vi "ProfilerTest.vi"() -> ()   [LabVIEW 2014] (continued)
"delVelocity"=0.0}, {"Time"=19.800000000000296, "delVelocity"=0.0}, {"Time"=19.810000000000297, "delVelocity"=0.0}, {"Time"=19.8200000000003, "delVelocity"=0.0}, {"Time"=19.8300000000003, "delVelocity"=0.0}, {"Time"=19.840000000000302, "delVelocity"=0.0}, {"Time"=19.850000000000303, "delVelocity"=0.0}, {"Time"=19.860000000000305, "delVelocity"=0.0}, {"Time"=19.870000000000307, "delVelocity"=0.0}, {"Time"=19.880000000000308, "delVelocity"=0.0}, {"Time"=19.89000000000031, "delVelocity"=0.0}, {"Time"=19.90000000000031, "delVelocity"=0.0}, {"Time"=19.910000000000313, "delVelocity"=0.0}, {"Time"=19.920000000000314, "delVelocity"=0.0}, {"Time"=19.930000000000316, "delVelocity"=0.0}, {"Time"=19.940000000000317, "delVelocity"=0.0}, {"Time"=19.95000000000032, "delVelocity"=0.0}, {"Time"=19.96000000000032, "delVelocity"=0.0}, {"Time"=19.970000000000322, "delVelocity"=0.0}, {"Time"=19.980000000000324, "delVelocity"=0.0}, {"Time"=19.990000000000325, "delVelocity"=0.0}, {"Time"=20.000000000000327, "delVelocity"=0.0}, {"Time"=20.01000000000033, "delVelocity"=0.0}, {"Time"=20.02000000000033, "delVelocity"=0.0}, {"Time"=20.03000000000033, "delVelocity"=0.0}, {"Time"=20.040000000000333, "delVelocity"=0.0}, {"Time"=20.050000000000335, "delVelocity"=0.0}, {"Time"=20.060000000000336, "delVelocity"=0.0}, {"Time"=20.070000000000338, "delVelocity"=0.0}, {"Time"=20.08000000000034, "delVelocity"=0.0}, {"Time"=20.09000000000034, "delVelocity"=0.0}, {"Time"=20.100000000000342, "delVelocity"=0.0}, {"Time"=20.110000000000344, "delVelocity"=0.0}, {"Time"=20.120000000000346, "delVelocity"=0.0}, {"Time"=20.130000000000347, "delVelocity"=0.0}, {"Time"=20.14000000000035, "delVelocity"=0.0}, {"Time"=20.15000000000035, "delVelocity"=0.0}, {"Time"=20.160000000000352, "delVelocity"=0.0}, {"Time"=20.170000000000353, "delVelocity"=0.0}, {"Time"=20.180000000000355, "delVelocity"=0.0}, {"Time"=20.190000000000357, "delVelocity"=0.0}, {"Time"=20.200000000000358, "delVelocity"=0.0}, {"Time"=20.21000000000036, "delVelocity"=0.0}, {"Time"=20.22000000000036, "delVelocity"=0.0}, {"Time"=20.230000000000363, "delVelocity"=0.0}, {"Time"=20.240000000000364, "delVelocity"=0.0}, {"Time"=20.250000000000366, "delVelocity"=0.0}, {"Time"=20.260000000000367, "delVelocity"=0.0}, {"Time"=20.27000000000037, "delVelocity"=0.0}, {"Time"=20.28000000000037, "delVelocity"=0.0}, {"Time"=20.290000000000372, "delVelocity"=0.0}, {"Time"=20.300000000000374, "delVelocity"=0.0}, {"Time"=20.310000000000375, "delVelocity"=0.0}, {"Time"=20.320000000000377, "delVelocity"=0.0}, {"Time"=20.33000000000038, "delVelocity"=0.0}, {"Time"=20.34000000000038, "delVelocity"=0.0}, {"Time"=20.35000000000038, "delVelocity"=0.0}, {"Time"=20.360000000000383, "delVelocity"=0.0}, {"Time"=20.370000000000385, "delVelocity"=0.0}, {"Time"=20.380000000000386, "delVelocity"=0.0}, {"Time"=20.390000000000388, "delVelocity"=0.0}, {"Time"=20.40000000000039, "delVelocity"=0.0}, {"Time"=20.41000000000039, "delVelocity"=0.0}, {"Time"=20.420000000000393, "delVelocity"=0.0}, {"Time"=20.430000000000394, "delVelocity"=0.0}, {"Time"=20.440000000000396, "delVelocity"=0.0}, {"Time"=20.450000000000397, "delVelocity"=0.0}, {"Time"=20.4600000000004, "delVelocity"=0.0}, {"Time"=20.4700000000004, "delVelocity"=0.0}, {"Time"=20.480000000000402, "delVelocity"=0.0}, {"Time"=20.490000000000403, "delVelocity"=0.0}, {"Time"=20.500000000000405, "delVelocity"=0.0}, {"Time"=20.510000000000407, "delVelocity"=0.0}, {"Time"=20.520000000000408, "delVelocity"=0.0}, {"Time"=20.53000000000041, "delVelocity"=0.0}, {"Time"=20.54000000000041, "delVelocity"=0.0}, {"Time"=20.550000000000413, "delVelocity"=0.0}, {"Time"=20.560000000000414, "delVelocity"=0.0}, {"Time"=20.570000000000416, "delVelocity"=0.0}, {"Time"=20.580000000000418, "delVelocity"=0.0}, {"Time"=20.59000000000042, "delVelocity"=0.0}, {"Time"=20.60000000000042, "delVelocity"=0.0}, {"Time"=20.610000000000422, "delVelocity"=0.0}, {"Time"=20.620000000000424, "delVelocity"=0.0}, {"Time"=20.630000000000425, "delVelocity"=0.0}, {"Time"=20.640000000000427, "delVelocity"=0.0}, {"Time"=20.65000000000043, "delVelocity"=0.0}, {"Time"=20.66000000000043, "delVelocity"=0.0}, {"Time"=20.67000000000043, "delVelocity"=0.0}, {"Time"=20.680000000000433, "delVelocity"=0.0}, {"Time"=20.690000000000435, "delVelocity"=0.0}, {"Time"=20.700000000000436, "delVelocity"=0.0}, {"Time"=20.710000000000438, "delVelocity"=0.0}, {"Time"=20.72000000000044, "delVelocity"=0.0}, {"Time"=20.73000000000044, "delVelocity"=0.0}, {"Time"=20.740000000000443, "delVelocity"=0.0}, {"Time"=20.750000000000444, "delVelocity"=0.0}, {"Time"=20.760000000000446, "delVelocity"=0.0}, {"Time"=20.770000000000447, "delVelocity"=0.0}, {"Time"=20.78000000000045, "delVelocity"=0.0}, {"Time"=20.79000000000045, "delVelocity"=0.0}, {"Time"=20.800000000000452, "delVelocity"=0.0}, {"Time"=20.810000000000453, "delVelocity"=0.0}, {"Time"=20.820000000000455, "delVelocity"=0.0}, {"Time"=20.830000000000457, "delVelocity"=0.0}, {"Time"=20.840000000000458, "delVelocity"=0.0}, {"Time"=20.85000000000046, "delVelocity"=0.0}, {"Time"=20.86000000000046, "delVelocity"=0.0}, {"Time"=20.870000000000463, "delVelocity"=0.0}, {"Time"=20.880000000000464, "delVelocity"=0.0}, {"Time"=20.890000000000466, "delVelocity"=0.0}, {"Time"=20.900000000000468, "delVelocity"=0.0}, {"Time"=20.91000000000047, "delVelocity"=0.0}, {"Time"=20.92000000000047, "delVelocity"=0.0}, {"Time"=20.930000000000472, "delVelocity"=0.0}, {"Time"=20.940000000000474, "delVelocity"=0.0}, {"Time"=20.950000000000475, "delVelocity"=0.0}, {"Time"=20.960000000000477, "delVelocity"=0.0}, {"Time"=20.97000000000048, "delVelocity"=0.0}, {"Time"=20.98000000000048, "delVelocity"=0.0}, {"Time"=20.99000000000048, "delVelocity"=0.0}, {"Time"=21.000000000000483, "delVelocity"=0.0}, {"Time"=21.010000000000485, "delVelocity"=0.0}, {"Time"=21.020000000000486, "delVelocity"=0.0}, {"Time"=21.030000000000488, "delVelocity"=0.0}, {"Time"=21.04000000000049, "delVelocity"=0.0}, {"Time"=21.05000000000049, "delVelocity"=0.0}, {"Time"=21.060000000000493, "delVelocity"=0.0}, {"Time"=21.070000000000494, "delVelocity"=0.0}, {"Time"=21.080000000000496, "delVelocity"=0.0}, {"Time"=21.090000000000497, "delVelocity"=0.0}, {"Time"=21.1000000000005, "delVelocity"=0.0}, {"Time"=21.1100000000005, "delVelocity"=0.0}, {"Time"=21.120000000000502, "delVelocity"=0.0}, {"Time"=21.130000000000503, "delVelocity"=0.0}, {"Time"=21.140000000000505, "delVelocity"=0.0}, {"Time"=21.150000000000507, "delVelocity"=0.0}, {"Time"=21.160000000000508, "delVelocity"=0.0}, {"Time"=21.17000000000051, "delVelocity"=0.0}, {"Time"=21.18000000000051, "delVelocity"=0.0}, {"Time"=21.190000000000513, "delVelocity"=0.0}, {"Time"=21.200000000000514, "delVelocity"=0.0}, {"Time"=21.210000000000516, "delVelocity"=0.0}, {"Time"=21.220000000000518, "delVelocity"=0.0}, {"Time"=21.23000000000052, "delVelocity"=0.0}, {"Time"=21.24000000000052, "delVelocity"=0.0}, {"Time"=21.250000000000522, "delVelocity"=0.0}, {"Time"=21.260000000000524, "delVelocity"=0.0}, {"Time"=21.270000000000525, "delVelocity"=0.0}, {"Time"=21.280000000000527, "delVelocity"=0.0}, {"Time"=21.29000000000053, "delVelocity"=0.0}, {"Time"=21.30000000000053, "delVelocity"=0.0}, {"Time"=21.31000000000053, "delVelocity"=0.0}, {"Time"=21.320000000000533, "delVelocity"=0.0}, {"Time"=21.330000000000535, "delVelocity"=0.0}, {"Time"=21.340000000000536, "delVelocity"=0.0}, {"Time"=21.350000000000538, "delVelocity"=0.0}, {"Time"=21.36000000000054, "delVelocity"=0.0}, {"Time"=21.37000000000054, "delVelocity"=0.0}, {"Time"=21.380000000000543, "delVelocity"=0.0}, {"Time"=21.390000000000544, "delVelocity"=0.0}, {"Time"=21.400000000000546, "delVelocity"=0.0}, {"Time"=21.410000000000547, "delVelocity"=0.0}, {"Time"=21.42000000000055, "delVelocity"=0.0}, {"Time"=21.43000000000055, "delVelocity"=0.0}, {"Time"=21.440000000000552, "delVelocity"=0.0}, {"Time"=21.450000000000554, "delVelocity"=0.0}, {"Time"=21.460000000000555, "delVelocity"=0.0}, {"Time"=21.470000000000557, "delVelocity"=0.0}, {"Time"=21.480000000000558, "delVelocity"=0.0}, {"Time"=21.49000000000056, "delVelocity"=0.0}, {"Time"=21.50000000000056, "delVelocity"=0.0}, {"Time"=21.510000000000563, "delVelocity"=0.0}, {"Time"=21.520000000000564, "delVelocity"=0.0}, {"Time"=21.530000000000566, "delVelocity"=0.0}, {"Time"=21.540000000000568, "delVelocity"=0.0}, {"Time"=21.55000000000057, "delVelocity"=0.0}, {"Time"=21.56000000000057, "delVelocity"=0.0}, {"Time"=21.570000000000572, "delVelocity"=0.0}, {"Time"=21.580000000000574, "delVelocity"=0.0}, {"Time"=21.590000000000575, "delVelocity"=0.0}, {"Time"=21.600000000000577, "delVelocity"=0.0}, {"Time"=21.61000000000058, "delVelocity"=0.0}, {"Time"=21.62000000000058, "delVelocity"=0.0}, {"Time"=21.63000000000058, "delVelocity"=0.0}, {"Time"=21.640000000000583, "delVelocity"=0.0}, {"Time"=21.650000000000585, "delVelocity"=0.0}, {"Time"=21.660000000000586, "delVelocity"=0.0}, {"Time"=21.670000000000588, "delVelocity"=0.0}, {"Time"=21.68000000000059, "delVelocity"=0.0}, {"Time"=21.69000000000059, "delVelocity"=0.0}, {"Time"=21.700000000000593, "delVelocity"=0.0}, {"Time"=21.710000000000594, "delVelocity"=0.0}, {"Time"=21.720000000000596, "delVelocity"=0.0}, {"Time"=21.730000000000597, "delVelocity"=0.0}, {"Time"=21.7400000000006, "delVelocity"=0.0}, {"Time"=21.7500000000006, "delVelocity"=0.0}, {"Time"=21.760000000000602, "delVelocity"=0.0}, {"Time"=21.770000000000604, "delVelocity"=0.0}, {"Time"=21.780000000000605, "delVelocity"=0.0}, {"Time"=21.790000000000607, "delVelocity"=0.0}, {"Time"=21.80000000000061, "delVelocity"=0.0}, {"Time"=21.81000000000061, "delVelocity"=0.0}, {"Time"=21.82000000000061, "delVelocity"=0.0}, {"Time"=21.830000000000613, "delVelocity"=0.0}, {"Time"=21.840000000000614, "delVelocity"=0.0}, {"Time"=21.850000000000616, "delVelocity"=0.0}, {"Time"=21.860000000000618, "delVelocity"=0.0}, {"Time"=21.87000000000062, "delVelocity"=0.0}, {"Time"=21.88000000000062, "delVelocity"=0.0}, {"Time"=21.890000000000622, "delVelocity"=0.0}, {"Time"=21.900000000000624, "delVelocity"=0.0}, {"Time"=21.910000000000625, "delVelocity"=0.0}, {"Time"=21.920000000000627, "delVelocity"=0.0}, {"Time"=21.93000000000063, "delVelocity"=0.0}, {"Time"=21.94000000000063, "delVelocity"=0.0}, {"Time"=21.95000000000063, "delVelocity"=0.0}, {"Time"=21.960000000000633, "delVelocity"=0.0}, {"Time"=21.970000000000635, "delVelocity"=0.0}, {"Time"=21.980000000000636, "delVelocity"=0.0}, {"Time"=21.990000000000638, "delVelocity"=0.0}, {"Time"=22.00000000000064, "delVelocity"=0.0}, {"Time"=22.01000000000064, "delVelocity"=0.0}, {"Time"=22.020000000000643, "delVelocity"=0.0}, {"Time"=22.030000000000644, "delVelocity"=0.0}, {"Time"=22.040000000000646, "delVelocity"=0.0}, {"Time"=22.050000000000647, "delVelocity"=0.0}, {"Time"=22.06000000000065, "delVelocity"=0.0}, {"Time"=22.07000000000065, "delVelocity"=0.0}, {"Time"=22.080000000000652, "delVelocity"=0.0}, {"Time"=22.090000000000654, "delVelocity"=0.0}, {"Time"=22.100000000000655, "delVelocity"=0.0}, {"Time"=22.110000000000657, "delVelocity"=0.0}, {"Time"=22.12000000000066, "delVelocity"=0.0}, {"Time"=22.13000000000066, "delVelocity"=0.0}, {"Time"=22.14000000000066, "delVelocity"=0.0}, {"Time"=22.150000000000663, "delVelocity"=0.0}, {"Time"=22.160000000000664, "delVelocity"=0.0}, {"Time"=22.170000000000666, "delVelocity"=0.0}, {"Time"=22.180000000000668, "delVelocity"=0.0}, {"Time"=22.19000000000067, "delVelocity"=0.0}, {"Time"=22.20000000000067, "delVelocity"=0.0}, {"Time"=22.210000000000672, "delVelocity"=0.0}, {"Time"=22.220000000000674, "delVelocity"=0.0}, {"Time"=22.230000000000675, "delVelocity"=0.0}, {"Time"=22.240000000000677, "delVelocity"=0.0}, {"Time"=22.25000000000068, "delVelocity"=0.0}, {"Time"=22.26000000000068, "delVelocity"=0.0}, {"Time"=22.27000000000068, "delVelocity"=0.0}, {"Time"=22.280000000000683, "delVelocity"=0.0}, {"Time"=22.290000000000685, "delVelocity"=0.0}, {"Time"=22.300000000000686, "delVelocity"=0.0}, {"Time"=22.310000000000688, "delVelocity"=0.0}, {"Time"=22.32000000000069, "delVelocity"=0.0}, {"Time"=22.33000000000069, "delVelocity"=0.0}, {"Time"=22.340000000000693, "delVelocity"=0.0}, {"Time"=22.350000000000694, "delVelocity"=0.0}, {"Time"=22.360000000000696, "delVelocity"=0.0}, {"Time"=22.370000000000697, "delVelocity"=0.0}, {"Time"=22.3800000000007, "delVelocity"=0.0}, {"Time"=22.3900000000007, "delVelocity"=0.0}, {"Time"=22.400000000000702, "delVelocity"=0.0}, {"Time"=22.410000000000704, "delVelocity"=0.0}, {"Time"=22.420000000000705, "delVelocity"=0.0}, {"Time"=22.430000000000707, "delVelocity"=0.0}, {"Time"=22.44000000000071, "delVelocity"=0.0}, {"Time"=22.45000000000071, "delVelocity"=0.0}, {"Time"=22.46000000000071, "delVelocity"=0.0}, {"Time"=22.470000000000713, "delVelocity"=0.0}, {"Time"=22.480000000000715, "delVelocity"=0.0}, {"Time"=22.490000000000716, "delVelocity"=0.0}, {"Time"=22.500000000000718, "delVelocity"=0.0}, {"Time"=22.51000000000072, "delVelocity"=0.0}, {"Time"=22.52000000000072, "delVelocity"=0.0}, {"Time"=22.530000000000722, "delVelocity"=0.0}, {"Time"=22.540000000000724, "delVelocity"=0.0}, {"Time"=22.550000000000725, "delVelocity"=0.0}, {"Time"=22.560000000000727, "delVelocity"=0.0}, {"Time"=22.57000000000073, "delVelocity"=0.0}, {"Time"=22.58000000000073, "delVelocity"=0.0}, {"Time"=22.59000000000073, "delVelocity"=0.0}, {"Time"=22.600000000000733, "delVelocity"=0.0}, {"Time"=22.610000000000735, "delVelocity"=0.0}, {"Time"=22.620000000000736, "delVelocity"=0.0}, {"Time"=22.630000000000738, "delVelocity"=0.0}, {"Time"=22.64000000000074, "delVelocity"=0.0}, {"Time"=22.65000000000074, "delVelocity"=0.0}, {"Time"=22.660000000000743, "delVelocity"=0.0}, {"Time"=22.670000000000744, "delVelocity"=0.0}, {"Time"=22.680000000000746, "delVelocity"=0.0}, {"Time"=22.690000000000747, "delVelocity"=0.0}, {"Time"=22.70000000000075, "delVelocity"=0.0}, {"Time"=22.71000000000075, "delVelocity"=0.0}, {"Time"=22.720000000000752, "delVelocity"=0.0}, {"Time"=22.730000000000754, "delVelocity"=0.0}, {"Time"=22.740000000000755, "delVelocity"=0.0}, {"Time"=22.750000000000757, "delVelocity"=0.0}, {"Time"=22.76000000000076, "delVelocity"=0.0}, {"Time"=22.77000000000076, "delVelocity"=0.0}, {"Time"=22.78000000000076, "delVelocity"=0.0}, {"Time"=22.790000000000763, "delVelocity"=0.0}, {"Time"=22.800000000000765, "delVelocity"=0.0}, {"Time"=22.810000000000766, "delVelocity"=0.0}, {"Time"=22.820000000000768, "delVelocity"=0.0}, {"Time"=22.83000000000077, "delVelocity"=0.0}, {"Time"=22.84000000000077, "delVelocity"=0.0}, {"Time"=22.850000000000772, "delVelocity"=0.0}, {"Time"=22.860000000000774, "delVelocity"=0.0}, {"Time"=22.870000000000775, "delVelocity"=0.0}, {"Time"=22.880000000000777, "delVelocity"=0.0}, {"Time"=22.89000000000078, "delVelocity"=0.0}, {"Time"=22.90000000000078, "delVelocity"=0.0}, {"Time"=22.91000000000078, "delVelocity"=0.0}, {"Time"=22.920000000000783, "delVelocity"=0.0}, {"Time"=22.930000000000785, "delVelocity"=0.0}, {"Time"=22.940000000000786, "delVelocity"=0.0}, {"Time"=22.950000000000788, "delVelocity"=0.0}, {"Time"=22.96000000000079, "delVelocity"=0.0}, {"Time"=22.97000000000079, "delVelocity"=0.0}, {"Time"=22.980000000000793, "delVelocity"=0.0}, {"Time"=22.990000000000794, "delVelocity"=0.0}, {"Time"=23.000000000000796, "delVelocity"=0.0}, {"Time"=23.010000000000797, "delVelocity"=0.0}, {"Time"=23.0200000000008, "delVelocity"=0.0}, {"Time"=23.0300000000008, "delVelocity"=0.0}, {"Time"=23.040000000000802, "delVelocity"=0.0}, {"Time"=23.050000000000804, "delVelocity"=0.0}, {"Time"=23.060000000000805, "delVelocity"=0.0}, {"Time"=23.070000000000807, "delVelocity"=0.0}, {"Time"=23.08000000000081, "delVelocity"=0.0}, {"Time"=23.09000000000081, "delVelocity"=0.0}, {"Time"=23.10000000000081, "delVelocity"=0.0}, {"Time"=23.110000000000813, "delVelocity"=0.0}, {"Time"=23.120000000000815, "delVelocity"=0.0}, {"Time"=23.130000000000816, "delVelocity"=0.0}, {"Time"=23.140000000000818, "delVelocity"=0.0}, {"Time"=23.15000000000082, "delVelocity"=0.0}, {"Time"=23.16000000000082, "delVelocity"=0.0}, {"Time"=23.170000000000822, "delVelocity"=0.0}, {"Time"=23.180000000000824, "delVelocity"=0.0}, {"Time"=23.190000000000826, "delVelocity"=0.0}, {"Time"=23.200000000000827, "delVelocity"=0.0}, {"Time"=23.21000000000083, "delVelocity"=0.0}, {"Time"=23.22000000000083, "delVelocity"=0.0}, {"Time"=23.23000000000083, "delVelocity"=0.0}, {"Time"=23.240000000000833, "delVelocity"=0.0}, {"Time"=23.250000000000835, "delVelocity"=0.0}, {"Time"=23.260000000000836, "delVelocity"=0.0}, {"Time"=23.270000000000838, "delVelocity"=0.0}, {"Time"=23.28000000000084, "delVelocity"=0.0}, {"Time"=23.29000000000084, "delVelocity"=0.0}, {"Time"=23.300000000000843, "delVelocity"=0.0}, {"Time"=23.310000000000844, "delVelocity"=0.0}, {"Time"=23.320000000000846, "delVelocity"=0.0}, {"Time"=23.330000000000847, "delVelocity"=0.0}, {"Time"=23.34000000000085, "delVelocity"=0.0}, {"Time"=23.35000000000085, "delVelocity"=0.0}, {"Time"=23.360000000000852, "delVelocity"=0.0}, {"Time"=23.370000000000854, "delVelocity"=0.0}, {"Time"=23.380000000000855, "delVelocity"=0.0}, {"Time"=23.390000000000857, "delVelocity"=0.0}, {"Time"=23.40000000000086, "delVelocity"=0.0}, {"Time"=23.41000000000086, "delVelocity"=0.0}, {"Time"=23.42000000000086, "delVelocity"=0.0}, {"Time"=23.430000000000863, "delVelocity"=0.0}, {"Time"=23.440000000000865, "delVelocity"=0.0}, {"Time"=23.450000000000866, "delVelocity"=0.0}, {"Time"=23.460000000000868, "delVelocity"=0.0}, {"Time"=23.47000000000087, "delVelocity"=0.0}, {"Time"=23.48000000000087, "delVelocity"=0.0}, {"Time"=23.490000000000872, "delVelocity"=0.0}, {"Time"=23.500000000000874, "delVelocity"=0.0}, {"Time"=23.510000000000876, "delVelocity"=0.0}, {"Time"=23.520000000000877, "delVelocity"=0.0}, {"Time"=23.53000000000088, "delVelocity"=0.0}, {"Time"=23.54000000000088, "delVelocity"=0.0}, {"Time"=23.550000000000882, "delVelocity"=0.0}, {"Time"=23.560000000000883, "delVelocity"=0.0}, {"Time"=23.570000000000885, "delVelocity"=0.0}, {"Time"=23.580000000000886, "delVelocity"=0.0}, {"Time"=23.590000000000888, "delVelocity"=0.0}, {"Time"=23.60000000000089, "delVelocity"=0.0}, {"Time"=23.61000000000089, "delVelocity"=0.0}, {"Time"=23.620000000000893, "delVelocity"=0.0}, {"Time"=23.630000000000894, "delVelocity"=0.0}, {"Time"=23.640000000000896, "delVelocity"=0.0}, {"Time"=23.650000000000897, "delVelocity"=0.0}, {"Time"=23.6600000000009, "delVelocity"=0.0}, {"Time"=23.6700000000009, "delVelocity"=0.0}, {"Time"=23.680000000000902, "delVelocity"=0.0}, {"Time"=23.690000000000904, "delVelocity"=0.0}, {"Time"=23.700000000000905, "delVelocity"=0.0}, {"Time"=23.710000000000907, "delVelocity"=0.0}, {"Time"=23.72000000000091, "delVelocity"=0.0}, {"Time"=23.73000000000091, "delVelocity"=0.0}, {"Time"=23.74000000000091, "delVelocity"=0.0}, {"Time"=23.750000000000913, "delVelocity"=0.0}, {"Time"=23.760000000000915, "delVelocity"=0.0}, {"Time"=23.770000000000916, "delVelocity"=0.0}, {"Time"=23.780000000000918, "delVelocity"=0.0}, {"Time"=23.79000000000092, "delVelocity"=0.0}, {"Time"=23.80000000000092, "delVelocity"=0.0}, {"Time"=23.810000000000922, "delVelocity"=0.0}, {"Time"=23.820000000000924, "delVelocity"=0.0}, {"Time"=23.830000000000926, "delVelocity"=0.0}, {"Time"=23.840000000000927, "delVelocity"=0.0}, {"Time"=23.85000000000093, "delVelocity"=0.0}, {"Time"=23.86000000000093, "delVelocity"=0.0}, {"Time"=23.870000000000932, "delVelocity"=0.0}, {"Time"=23.880000000000933, "delVelocity"=0.0}, {"Time"=23.890000000000935, "delVelocity"=0.0}, {"Time"=23.900000000000936, "delVelocity"=0.0}, {"Time"=23.910000000000938, "delVelocity"=0.0}, {"Time"=23.92000000000094, "delVelocity"=0.0}, {"Time"=23.93000000000094, "delVelocity"=0.0}, {"Time"=23.940000000000943, "delVelocity"=0.0}, {"Time"=23.950000000000944, "delVelocity"=0.0}, {"Time"=23.960000000000946, "delVelocity"=0.0}, {"Time"=23.970000000000947, "delVelocity"=0.0}, {"Time"=23.98000000000095, "delVelocity"=0.0}, {"Time"=23.99000000000095, "delVelocity"=0.0}, {"Time"=24.000000000000952, "delVelocity"=0.0}, {"Time"=24.010000000000954, "delVelocity"=0.0}, {"Time"=24.020000000000955, "delVelocity"=0.0}, {"Time"=24.030000000000957, "delVelocity"=0.0}, {"Time"=24.04000000000096, "delVelocity"=0.0}, {"Time"=24.05000000000096, "delVelocity"=0.0}, {"Time"=24.06000000000096, "delVelocity"=0.0}, {"Time"=24.070000000000963, "delVelocity"=0.0}, {"Time"=24.080000000000965, "delVelocity"=0.0}, {"Time"=24.090000000000966, "delVelocity"=0.0}, {"Time"=24.100000000000968, "delVelocity"=0.0}, {"Time"=24.11000000000097, "delVelocity"=0.0}, {"Time"=24.12000000000097, "delVelocity"=0.0}, {"Time"=24.130000000000972, "delVelocity"=0.0}, {"Time"=24.140000000000974, "delVelocity"=0.0}, {"Time"=24.150000000000976, "delVelocity"=0.0}, {"Time"=24.160000000000977, "delVelocity"=0.0}, {"Time"=24.17000000000098, "delVelocity"=0.0}, {"Time"=24.18000000000098, "delVelocity"=0.0}, {"Time"=24.190000000000982, "delVelocity"=0.0}, {"Time"=24.200000000000983, "delVelocity"=0.0}, {"Time"=24.210000000000985, "delVelocity"=0.0}, {"Time"=24.220000000000987, "delVelocity"=0.0}, {"Time"=24.230000000000988, "delVelocity"=0.0}, {"Time"=24.24000000000099, "delVelocity"=0.0}, {"Time"=24.25000000000099, "delVelocity"=0.0}, {"Time"=24.260000000000993, "delVelocity"=0.0}, {"Time"=24.270000000000994, "delVelocity"=0.0}, {"Time"=24.280000000000996, "delVelocity"=0.0}, {"Time"=24.290000000000997, "delVelocity"=0.0}, {"Time"=24.300000000001, "delVelocity"=0.0}, {"Time"=24.310000000001, "delVelocity"=0.0}, {"Time"=24.320000000001002, "delVelocity"=0.0}, {"Time"=24.330000000001004, "delVelocity"=0.0}, {"Time"=24.340000000001005, "delVelocity"=0.0}, {"Time"=24.350000000001007, "delVelocity"=0.0}, {"Time"=24.36000000000101, "delVelocity"=0.0}, {"Time"=24.37000000000101, "delVelocity"=0.0}, {"Time"=24.38000000000101, "delVelocity"=0.0}, {"Time"=24.390000000001013, "delVelocity"=0.0}, {"Time"=24.400000000001015, "delVelocity"=0.0}, {"Time"=24.410000000001016, "delVelocity"=0.0}, {"Time"=24.420000000001018, "delVelocity"=0.0}, {"Time"=24.43000000000102, "delVelocity"=0.0}, {"Time"=24.44000000000102, "delVelocity"=0.0}, {"Time"=24.450000000001022, "delVelocity"=0.0}, {"Time"=24.460000000001024, "delVelocity"=0.0}, {"Time"=24.470000000001026, "delVelocity"=0.0}, {"Time"=24.480000000001027, "delVelocity"=0.0}, {"Time"=24.49000000000103, "delVelocity"=0.0}, {"Time"=24.50000000000103, "delVelocity"=0.0}, {"Time"=24.510000000001032, "delVelocity"=0.0}, {"Time"=24.520000000001033, "delVelocity"=0.0}, {"Time"=24.530000000001035, "delVelocity"=0.0}, {"Time"=24.540000000001037, "delVelocity"=0.0}, {"Time"=24.550000000001038, "delVelocity"=0.0}, {"Time"=24.56000000000104, "delVelocity"=0.0}, {"Time"=24.57000000000104, "delVelocity"=0.0}, {"Time"=24.580000000001043, "delVelocity"=0.0}, {"Time"=24.590000000001044, "delVelocity"=0.0}, {"Time"=24.600000000001046, "delVelocity"=0.0}, {"Time"=24.610000000001047, "delVelocity"=0.0}, {"Time"=24.62000000000105, "delVelocity"=0.0}, {"Time"=24.63000000000105, "delVelocity"=0.0}, {"Time"=24.640000000001052, "delVelocity"=0.0}, {"Time"=24.650000000001054, "delVelocity"=0.0}, {"Time"=24.660000000001055, "delVelocity"=0.0}, {"Time"=24.670000000001057, "delVelocity"=0.0}, {"Time"=24.68000000000106, "delVelocity"=0.0}, {"Time"=24.69000000000106, "delVelocity"=0.0}, {"Time"=24.70000000000106, "delVelocity"=0.0}, {"Time"=24.710000000001063, "delVelocity"=0.0}, {"Time"=24.720000000001065, "delVelocity"=0.0}, {"Time"=24.730000000001066, "delVelocity"=0.0}, {"Time"=24.740000000001068, "delVelocity"=0.0}, {"Time"=24.75000000000107, "delVelocity"=0.0}, {"Time"=24.76000000000107, "delVelocity"=0.0}, {"Time"=24.770000000001072, "delVelocity"=0.0}, {"Time"=24.780000000001074, "delVelocity"=0.0}, {"Time"=24.790000000001076, "delVelocity"=0.0}, {"Time"=24.800000000001077, "delVelocity"=0.0}, {"Time"=24.81000000000108, "delVelocity"=0.0}, {"Time"=24.82000000000108, "delVelocity"=0.0}, {"Time"=24.830000000001082, "delVelocity"=0.0}, {"Time"=24.840000000001083, "delVelocity"=0.0}, {"Time"=24.850000000001085, "delVelocity"=0.0}, {"Time"=24.860000000001087, "delVelocity"=0.0}, {"Time"=24.870000000001088, "delVelocity"=0.0}, {"Time"=24.88000000000109, "delVelocity"=0.0}, {"Time"=24.89000000000109, "delVelocity"=0.0}, {"Time"=24.900000000001093, "delVelocity"=0.0}, {"Time"=24.910000000001094, "delVelocity"=0.0}, {"Time"=24.920000000001096, "delVelocity"=0.0}, {"Time"=24.930000000001098, "delVelocity"=0.0}, {"Time"=24.9400000000011, "delVelocity"=0.0}, {"Time"=24.9500000000011, "delVelocity"=0.0}, {"Time"=24.960000000001102, "delVelocity"=0.0}, {"Time"=24.970000000001104, "delVelocity"=0.0}, {"Time"=24.980000000001105, "delVelocity"=0.0}, {"Time"=24.990000000001107, "delVelocity"=0.0}, {"Time"=25.00000000000111, "delVelocity"=0.0}, {"Time"=25.01000000000111, "delVelocity"=0.0}, {"Time"=25.02000000000111, "delVelocity"=0.0}, {"Time"=25.030000000001113, "delVelocity"=0.0}, {"Time"=25.040000000001115, "delVelocity"=0.0}, {"Time"=25.050000000001116, "delVelocity"=0.0}, {"Time"=25.060000000001118, "delVelocity"=0.0}, {"Time"=25.07000000000112, "delVelocity"=0.0}, {"Time"=25.08000000000112, "delVelocity"=0.0}, {"Time"=25.090000000001123, "delVelocity"=0.0}, {"Time"=25.100000000001124, "delVelocity"=0.0}, {"Time"=25.110000000001126, "delVelocity"=0.0}, {"Time"=25.120000000001127, "delVelocity"=0.0}, {"Time"=25.13000000000113, "delVelocity"=0.0}, {"Time"=25.14000000000113, "delVelocity"=0.0}, {"Time"=25.150000000001132, "delVelocity"=0.0}, {"Time"=25.160000000001133, "delVelocity"=0.0}, {"Time"=25.170000000001135, "delVelocity"=0.0}, {"Time"=25.180000000001137, "delVelocity"=0.0}, {"Time"=25.190000000001138, "delVelocity"=0.0}, {"Time"=25.20000000000114, "delVelocity"=0.0}, {"Time"=25.21000000000114, "delVelocity"=0.0}, {"Time"=25.220000000001143, "delVelocity"=0.0}, {"Time"=25.230000000001144, "delVelocity"=0.0}, {"Time"=25.240000000001146, "delVelocity"=0.0}, {"Time"=25.250000000001148, "delVelocity"=0.0}, {"Time"=25.26000000000115, "delVelocity"=0.0}, {"Time"=25.27000000000115, "delVelocity"=0.0}, {"Time"=25.280000000001152, "delVelocity"=0.0}, {"Time"=25.290000000001154, "delVelocity"=0.0}, {"Time"=25.300000000001155, "delVelocity"=0.0}, {"Time"=25.310000000001157, "delVelocity"=0.0}, {"Time"=25.32000000000116, "delVelocity"=0.0}, {"Time"=25.33000000000116, "delVelocity"=0.0}, {"Time"=25.34000000000116, "delVelocity"=0.0}, {"Time"=25.350000000001163, "delVelocity"=0.0}, {"Time"=25.360000000001165, "delVelocity"=0.0}, {"Time"=25.370000000001166, "delVelocity"=0.0}, {"Time"=25.380000000001168, "delVelocity"=0.0}, {"Time"=25.39000000000117, "delVelocity"=0.0}, {"Time"=25.40000000000117, "delVelocity"=0.0}, {"Time"=25.410000000001173, "delVelocity"=0.0}, {"Time"=25.420000000001174, "delVelocity"=0.0}, {"Time"=25.430000000001176, "delVelocity"=0.0}, {"Time"=25.440000000001177, "delVelocity"=0.0}, {"Time"=25.45000000000118, "delVelocity"=0.0}, {"Time"=25.46000000000118, "delVelocity"=0.0}, {"Time"=25.470000000001182, "delVelocity"=0.0}, {"Time"=25.480000000001183, "delVelocity"=0.0}, {"Time"=25.490000000001185, "delVelocity"=0.0}, {"Time"=25.500000000001187, "delVelocity"=0.0}, {"Time"=25.510000000001188, "delVelocity"=0.0}, {"Time"=25.52000000000119, "delVelocity"=0.0}, {"Time"=25.53000000000119, "delVelocity"=0.0}, {"Time"=25.540000000001193, "delVelocity"=0.0}, {"Time"=25.550000000001194, "delVelocity"=0.0}, {"Time"=25.560000000001196, "delVelocity"=0.0}, {"Time"=25.570000000001198, "delVelocity"=0.0}, {"Time"=25.5800000000012, "delVelocity"=0.0}, {"Time"=25.5900000000012, "delVelocity"=0.0}, {"Time"=25.600000000001202, "delVelocity"=0.0}, {"Time"=25.610000000001204, "delVelocity"=0.0}, {"Time"=25.620000000001205, "delVelocity"=0.0}, {"Time"=25.630000000001207, "delVelocity"=0.0}, {"Time"=25.64000000000121, "delVelocity"=0.0}, {"Time"=25.65000000000121, "delVelocity"=0.0}, {"Time"=25.66000000000121, "delVelocity"=0.0}, {"Time"=25.670000000001213, "delVelocity"=0.0}, {"Time"=25.680000000001215, "delVelocity"=0.0}, {"Time"=25.690000000001216, "delVelocity"=0.0}, {"Time"=25.700000000001218, "delVelocity"=0.0}, {"Time"=25.71000000000122, "delVelocity"=0.0}, {"Time"=25.72000000000122, "delVelocity"=0.0}, {"Time"=25.730000000001223, "delVelocity"=0.0}, {"Time"=25.740000000001224, "delVelocity"=0.0}, {"Time"=25.750000000001226, "delVelocity"=0.0}, {"Time"=25.760000000001227, "delVelocity"=0.0}, {"Time"=25.77000000000123, "delVelocity"=0.0}, {"Time"=25.78000000000123, "delVelocity"=0.0}, {"Time"=25.790000000001232, "delVelocity"=0.0}, {"Time"=25.800000000001234, "delVelocity"=0.0}, {"Time"=25.810000000001235, "delVelocity"=0.0}, {"Time"=25.820000000001237, "delVelocity"=0.0}, {"Time"=25.830000000001238, "delVelocity"=0.0}, {"Time"=25.84000000000124, "delVelocity"=0.0}, {"Time"=25.85000000000124, "delVelocity"=0.0}, {"Time"=25.860000000001243, "delVelocity"=0.0}, {"Time"=25.870000000001244, "delVelocity"=0.0}, {"Time"=25.880000000001246, "delVelocity"=0.0}, {"Time"=25.890000000001248, "delVelocity"=0.0}, {"Time"=25.90000000000125, "delVelocity"=0.0}, {"Time"=25.91000000000125, "delVelocity"=0.0}, {"Time"=25.920000000001252, "delVelocity"=0.0}, {"Time"=25.930000000001254, "delVelocity"=0.0}, {"Time"=25.940000000001255, "delVelocity"=0.0}, {"Time"=25.950000000001257, "delVelocity"=0.0}, {"Time"=25.96000000000126, "delVelocity"=0.0}, {"Time"=25.97000000000126, "delVelocity"=0.0}, {"Time"=25.98000000000126, "delVelocity"=0.0}, {"Time"=25.990000000001263, "delVelocity"=0.0}, {"Time"=26.000000000001265, "delVelocity"=0.0}, {"Time"=26.010000000001266, "delVelocity"=0.0}, {"Time"=26.020000000001268, "delVelocity"=0.0}, {"Time"=26.03000000000127, "delVelocity"=0.0}, {"Time"=26.04000000000127, "delVelocity"=0.0}, {"Time"=26.050000000001273, "delVelocity"=0.0}, {"Time"=26.060000000001274, "delVelocity"=0.0}, {"Time"=26.070000000001276, "delVelocity"=0.0}, {"Time"=26.080000000001277, "delVelocity"=0.0}, {"Time"=26.09000000000128, "delVelocity"=0.0}, {"Time"=26.10000000000128, "delVelocity"=0.0}, {"Time"=26.110000000001282, "delVelocity"=0.0}, {"Time"=26.120000000001284, "delVelocity"=0.0}, {"Time"=26.130000000001285, "delVelocity"=0.0}, {"Time"=26.140000000001287, "delVelocity"=0.0}, {"Time"=26.150000000001288, "delVelocity"=0.0}, {"Time"=26.16000000000129, "delVelocity"=0.0}, {"Time"=26.17000000000129, "delVelocity"=0.0}, {"Time"=26.180000000001293, "delVelocity"=0.0}, {"Time"=26.190000000001294, "delVelocity"=0.0}, {"Time"=26.200000000001296, "delVelocity"=0.0}, {"Time"=26.210000000001298, "delVelocity"=0.0}, {"Time"=26.2200000000013, "delVelocity"=0.0}, {"Time"=26.2300000000013, "delVelocity"=0.0}, {"Time"=26.240000000001302, "delVelocity"=0.0}, {"Time"=26.250000000001304, "delVelocity"=0.0}, {"Time"=26.260000000001305, "delVelocity"=0.0}, {"Time"=26.270000000001307, "delVelocity"=0.0}, {"Time"=26.28000000000131, "delVelocity"=0.0}, {"Time"=26.29000000000131, "delVelocity"=0.0}, {"Time"=26.30000000000131, "delVelocity"=0.0}, {"Time"=26.310000000001313, "delVelocity"=0.0}, {"Time"=26.320000000001315, "delVelocity"=0.0}, {"Time"=26.330000000001316, "delVelocity"=0.0}, {"Time"=26.340000000001318, "delVelocity"=0.0}, {"Time"=26.35000000000132, "delVelocity"=0.0}, {"Time"=26.36000000000132, "delVelocity"=0.0}, {"Time"=26.370000000001323, "delVelocity"=0.0}, {"Time"=26.380000000001324, "delVelocity"=0.0}, {"Time"=26.390000000001326, "delVelocity"=0.0}, {"Time"=26.400000000001327, "delVelocity"=0.0}, {"Time"=26.41000000000133, "delVelocity"=0.0}, {"Time"=26.42000000000133, "delVelocity"=0.0}, {"Time"=26.430000000001332, "delVelocity"=0.0}, {"Time"=26.440000000001334, "delVelocity"=0.0}, {"Time"=26.450000000001335, "delVelocity"=0.0}, {"Time"=26.460000000001337, "delVelocity"=0.0}, {"Time"=26.47000000000134, "delVelocity"=0.0}, {"Time"=26.48000000000134, "delVelocity"=0.0}, {"Time"=26.49000000000134, "delVelocity"=0.0}, {"Time"=26.500000000001343, "delVelocity"=0.0}, {"Time"=26.510000000001344, "delVelocity"=0.0}, {"Time"=26.520000000001346, "delVelocity"=0.0}, {"Time"=26.530000000001348, "delVelocity"=0.0}, {"Time"=26.54000000000135, "delVelocity"=0.0}, {"Time"=26.55000000000135, "delVelocity"=0.0}, {"Time"=26.560000000001352, "delVelocity"=0.0}, {"Time"=26.570000000001354, "delVelocity"=0.0}, {"Time"=26.580000000001355, "delVelocity"=0.0}, {"Time"=26.590000000001357, "delVelocity"=0.0}, {"Time"=26.60000000000136, "delVelocity"=0.0}, {"Time"=26.61000000000136, "delVelocity"=0.0}, {"Time"=26.62000000000136, "delVelocity"=0.0}, {"Time"=26.630000000001363, "delVelocity"=0.0}, {"Time"=26.640000000001365, "delVelocity"=0.0}, {"Time"=26.650000000001366, "delVelocity"=0.0}, {"Time"=26.660000000001368, "delVelocity"=0.0}, {"Time"=26.67000000000137, "delVelocity"=0.0}, {"Time"=26.68000000000137, "delVelocity"=0.0}, {"Time"=26.690000000001373, "delVelocity"=0.0}, {"Time"=26.700000000001374, "delVelocity"=0.0}, {"Time"=26.710000000001376, "delVelocity"=0.0}, {"Time"=26.720000000001377, "delVelocity"=0.0}, {"Time"=26.73000000000138, "delVelocity"=0.0}, {"Time"=26.74000000000138, "delVelocity"=0.0}, {"Time"=26.750000000001382, "delVelocity"=0.0}, {"Time"=26.760000000001384, "delVelocity"=0.0}, {"Time"=26.770000000001385, "delVelocity"=0.0}, {"Time"=26.780000000001387, "delVelocity"=0.0}, {"Time"=26.79000000000139, "delVelocity"=0.0}, {"Time"=26.80000000000139, "delVelocity"=0.0}, {"Time"=26.81000000000139, "delVelocity"=0.0}, {"Time"=26.820000000001393, "delVelocity"=0.0}, {"Time"=26.830000000001395, "delVelocity"=0.0}, {"Time"=26.840000000001396, "delVelocity"=0.0}, {"Time"=26.850000000001398, "delVelocity"=0.0}, {"Time"=26.8600000000014, "delVelocity"=0.0}, {"Time"=26.8700000000014, "delVelocity"=0.0}, {"Time"=26.880000000001402, "delVelocity"=0.0}, {"Time"=26.890000000001404, "delVelocity"=0.0}, {"Time"=26.900000000001405, "delVelocity"=0.0}, {"Time"=26.910000000001407, "delVelocity"=0.0}, {"Time"=26.92000000000141, "delVelocity"=0.0}, {"Time"=26.93000000000141, "delVelocity"=0.0}, {"Time"=26.94000000000141, "delVelocity"=0.0}, {"Time"=26.950000000001413, "delVelocity"=0.0}, {"Time"=26.960000000001415, "delVelocity"=0.0}, {"Time"=26.970000000001416, "delVelocity"=0.0}, {"Time"=26.980000000001418, "delVelocity"=0.0}, {"Time"=26.99000000000142, "delVelocity"=0.0}, {"Time"=27.00000000000142, "delVelocity"=0.0}, {"Time"=27.010000000001423, "delVelocity"=0.0}, {"Time"=27.020000000001424, "delVelocity"=0.0}, {"Time"=27.030000000001426, "delVelocity"=0.0}, {"Time"=27.040000000001427, "delVelocity"=0.0}, {"Time"=27.05000000000143, "delVelocity"=0.0}, {"Time"=27.06000000000143, "delVelocity"=0.0}, {"Time"=27.070000000001432, "delVelocity"=0.0}, {"Time"=27.080000000001434, "delVelocity"=0.0}, {"Time"=27.090000000001435, "delVelocity"=0.0}, {"Time"=27.100000000001437, "delVelocity"=0.0}, {"Time"=27.11000000000144, "delVelocity"=0.0}, {"Time"=27.12000000000144, "delVelocity"=0.0}, {"Time"=27.13000000000144, "delVelocity"=0.0}, {"Time"=27.140000000001443, "delVelocity"=0.0}, {"Time"=27.150000000001445, "delVelocity"=0.0}, {"Time"=27.160000000001446, "delVelocity"=0.0}, {"Time"=27.170000000001448, "delVelocity"=0.0}, {"Time"=27.18000000000145, "delVelocity"=0.0}, {"Time"=27.19000000000145, "delVelocity"=0.0}, {"Time"=27.200000000001452, "delVelocity"=0.0}, {"Time"=27.210000000001454, "delVelocity"=0.0}, {"Time"=27.220000000001455, "delVelocity"=0.0}, {"Time"=27.230000000001457, "delVelocity"=0.0}, {"Time"=27.24000000000146, "delVelocity"=0.0}, {"Time"=27.25000000000146, "delVelocity"=0.0}, {"Time"=27.26000000000146, "delVelocity"=0.0}, {"Time"=27.270000000001463, "delVelocity"=0.0}, {"Time"=27.280000000001465, "delVelocity"=0.0}, {"Time"=27.290000000001466, "delVelocity"=0.0}, {"Time"=27.300000000001468, "delVelocity"=0.0}, {"Time"=27.31000000000147, "delVelocity"=0.0}, {"Time"=27.32000000000147, "delVelocity"=0.0}, {"Time"=27.330000000001473, "delVelocity"=0.0}, {"Time"=27.340000000001474, "delVelocity"=0.0}, {"Time"=27.350000000001476, "delVelocity"=0.0}, {"Time"=27.360000000001477, "delVelocity"=0.0}, {"Time"=27.37000000000148, "delVelocity"=0.0}, {"Time"=27.38000000000148, "delVelocity"=0.0}, {"Time"=27.390000000001482, "delVelocity"=0.0}, {"Time"=27.400000000001484, "delVelocity"=0.0}, {"Time"=27.410000000001485, "delVelocity"=0.0}, {"Time"=27.420000000001487, "delVelocity"=0.0}, {"Time"=27.43000000000149, "delVelocity"=0.0}, {"Time"=27.44000000000149, "delVelocity"=0.0}, {"Time"=27.45000000000149, "delVelocity"=0.0}, {"Time"=27.460000000001493, "delVelocity"=0.0}, {"Time"=27.470000000001495, "delVelocity"=0.0}, {"Time"=27.480000000001496, "delVelocity"=0.0}, {"Time"=27.490000000001498, "delVelocity"=0.0}, {"Time"=27.5000000000015, "delVelocity"=0.0}, {"Time"=27.5100000000015, "delVelocity"=0.0}, {"Time"=27.520000000001502, "delVelocity"=0.0}, {"Time"=27.530000000001504, "delVelocity"=0.0}, {"Time"=27.540000000001505, "delVelocity"=0.0}, {"Time"=27.550000000001507, "delVelocity"=0.0}, {"Time"=27.56000000000151, "delVelocity"=0.0}, {"Time"=27.57000000000151, "delVelocity"=0.0}, {"Time"=27.58000000000151, "delVelocity"=0.0}, {"Time"=27.590000000001513, "delVelocity"=0.0}, {"Time"=27.600000000001515, "delVelocity"=0.0}, {"Time"=27.610000000001516, "delVelocity"=0.0}, {"Time"=27.620000000001518, "delVelocity"=0.0}, {"Time"=27.63000000000152, "delVelocity"=0.0}, {"Time"=27.64000000000152, "delVelocity"=0.0}, {"Time"=27.650000000001523, "delVelocity"=0.0}, {"Time"=27.660000000001524, "delVelocity"=0.0}, {"Time"=27.670000000001526, "delVelocity"=0.0}, {"Time"=27.680000000001527, "delVelocity"=0.0}, {"Time"=27.69000000000153, "delVelocity"=0.0}, {"Time"=27.70000000000153, "delVelocity"=0.0}, {"Time"=27.710000000001532, "delVelocity"=0.0}, {"Time"=27.720000000001534, "delVelocity"=0.0}, {"Time"=27.730000000001535, "delVelocity"=0.0}, {"Time"=27.740000000001537, "delVelocity"=0.0}, {"Time"=27.75000000000154, "delVelocity"=0.0}, {"Time"=27.76000000000154, "delVelocity"=0.0}, {"Time"=27.77000000000154, "delVelocity"=0.0}, {"Time"=27.780000000001543, "delVelocity"=0.0}, {"Time"=27.790000000001545, "delVelocity"=0.0}, {"Time"=27.800000000001546, "delVelocity"=0.0}, {"Time"=27.810000000001548, "delVelocity"=0.0}, {"Time"=27.82000000000155, "delVelocity"=0.0}, {"Time"=27.83000000000155, "delVelocity"=0.0}, {"Time"=27.840000000001552, "delVelocity"=0.0}, {"Time"=27.850000000001554, "delVelocity"=0.0}, {"Time"=27.860000000001556, "delVelocity"=0.0}, {"Time"=27.870000000001557, "delVelocity"=0.0}, {"Time"=27.88000000000156, "delVelocity"=0.0}, {"Time"=27.89000000000156, "delVelocity"=0.0}, {"Time"=27.90000000000156, "delVelocity"=0.0}, {"Time"=27.910000000001563, "delVelocity"=0.0}, {"Time"=27.920000000001565, "delVelocity"=0.0}, {"Time"=27.930000000001566, "delVelocity"=0.0}, {"Time"=27.940000000001568, "delVelocity"=0.0}, {"Time"=27.95000000000157, "delVelocity"=0.0}, {"Time"=27.96000000000157, "delVelocity"=0.0}, {"Time"=27.970000000001573, "delVelocity"=0.0}, {"Time"=27.980000000001574, "delVelocity"=0.0}, {"Time"=27.990000000001576, "delVelocity"=0.0}, {"Time"=28.000000000001577, "delVelocity"=0.0}, {"Time"=28.01000000000158, "delVelocity"=0.0}, {"Time"=28.02000000000158, "delVelocity"=0.0}, {"Time"=28.030000000001582, "delVelocity"=0.0}, {"Time"=28.040000000001584, "delVelocity"=0.0}, {"Time"=28.050000000001585, "delVelocity"=0.0}, {"Time"=28.060000000001587, "delVelocity"=0.0}, {"Time"=28.07000000000159, "delVelocity"=0.0}, {"Time"=28.08000000000159, "delVelocity"=0.0}, {"Time"=28.09000000000159, "delVelocity"=0.0}, {"Time"=28.100000000001593, "delVelocity"=0.0}, {"Time"=28.110000000001595, "delVelocity"=0.0}, {"Time"=28.120000000001596, "delVelocity"=0.0}, {"Time"=28.130000000001598, "delVelocity"=0.0}, {"Time"=28.1400000000016, "delVelocity"=0.0}, {"Time"=28.1500000000016, "delVelocity"=0.0}, {"Time"=28.160000000001602, "delVelocity"=0.0}, {"Time"=28.170000000001604, "delVelocity"=0.0}, {"Time"=28.180000000001606, "delVelocity"=0.0}, {"Time"=28.190000000001607, "delVelocity"=0.0}, 
